vi "Encode TextString.vi"(10 "Text String":string) -> (3 "Length-Prefixed Field":u8[](array[numeric]) format="%08b")   [LabVIEW 2013, in "MQTT_Control_Packets.lvlib" / "ControlPacket.lvclass"]
uses:
  ControlPacket.lvclass
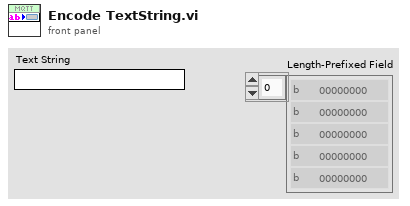
[diagram p1: front panel]
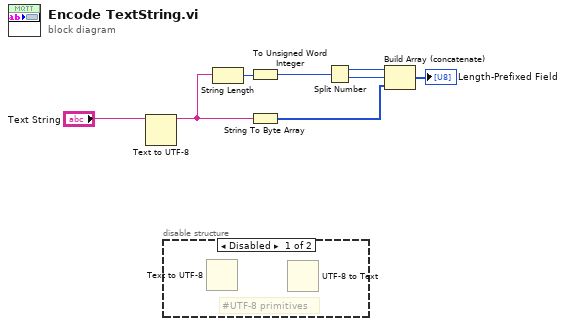
[diagram p0: block diagram]
diagram:
  n1 = Text to UTF-8(11:"Text String") -> (3:w4:string)  [unwired: 1 in, 1 out]
  n2 = disable-structure shown="Disabled" {
    frame Disabled {
      # "#UTF-8 primitives"
      n3 = Text to UTF-8() -> ()  [unwired: 2 in, 2 out]
      n4 = UTF-8 to Text() -> ()  [unwired: 2 in, 2 out]
    }
    frame Enabled {
    }
  }
  n5 = String Length(string=w4) -> (length=w7:i32)
  n6 = To Unsigned Word Integer(number=w7) -> (unsigned 16bit integer=w1:u16)
  n7 = String To Byte Array(string=w4) -> (unsigned byte array=w3:u8[])
  n8 = Split Number(x=w1) -> (hi(x)=w6:u8, lo(x)=w5:u8)
  n9 = Build Array (concatenate)(w6, w5, w3) -> (→"Length-Prefixed Field":u8[])
